vi "Acquire Data using Metronome - cRIO.vi"() -> ()   [LabVIEW 2010]
uses:
  <vilib>/eio/EIONode/EIONode.xnode
  <vilib>/rvi/eio/nirviEIOImplementation/nirviEIOImplementation.xnode
  <vilib>/rvi/eio/common/nirviEmuClasses.ctl
  <vilib>/rvi/eio/common/nirviEmuTemplateMethod_noerrors.vi
  FPGA Timekeeper.lvlib
panel:
  out "sample timestamp (ns)":u64
  out "Mod1/AI0":fxp<+/-,20,5>
  in  "loop period (ns)":u32=1000000000
  in  "start time (ns)":u64
  out "offset from time reference":i32
  out "FPGA Timekeeper locked":bool
  out "FPGA Timekeeper time (ns)":u64
  # "This example samples an analog input using the Metronome VI of the FPGA Timekeeper API."
  # "Analog Sampling Info"
  # "The default values for the controls  loop period (ns), and start time (ns) will sample an analog input at the rate of 1 Hz with each sample aligned to the beginning of each second."
  # "Acquired Data"
  # "Analog input modules need time to perform the conversion.  The difference in time between when the start of the conversion and the sample timestamp is the conversion time."
  # "FPGA Timekeeper"
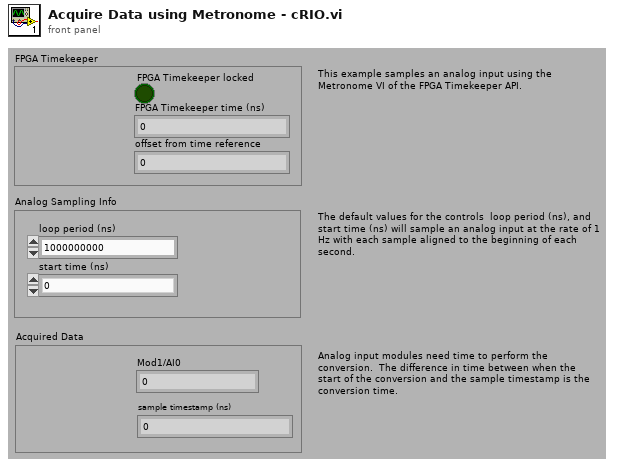
[diagram p1: front panel]
types:
  T1 = typedef "nirviEmuClasses.ctl" = enum16{"IO Read", "IO Write", "Method", "Property Read", "Property Write"}
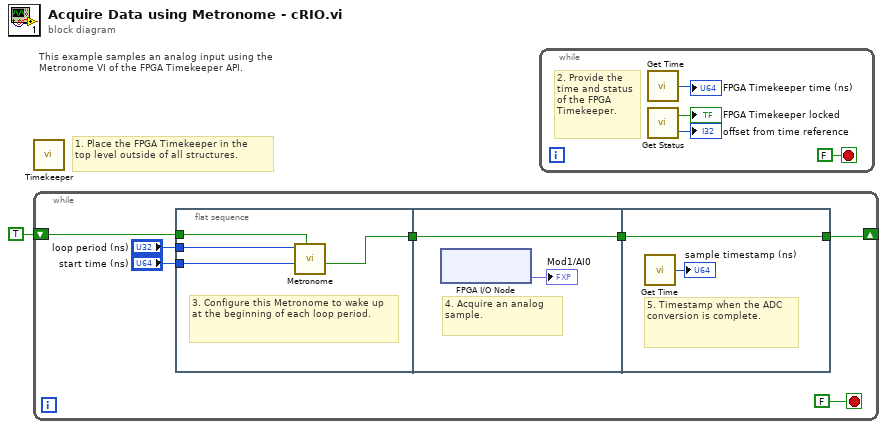
[diagram p0: block diagram]
diagram:
  # "This example samples an analog input using the Metronome VI of the FPGA Timekeeper API."
  # "1. Place the FPGA Timekeeper in the\ntop level outside of all structures."
  n1 = call "Timekeeper.vi"() -> ()  [unwired: 12 in]
  n2 = while {
    shift-right: [w7] -> _
    shift-left: TRUE ("Time Snapped Event") -> [w8]
    stop <- FALSE stop-if-true
    n3 = flat-sequence {
      tunnel: w8 -> [w12]
      tunnel: "start time (ns)" -> [w10]
      tunnel: "loop period (ns)" -> [w11]
      tunnel: [w9] -> w3
      tunnel: w3 -> [w14]
      tunnel: [w14] -> w2
      tunnel: [w35] -> w7
      tunnel: w2 -> [w35]
      frame #0 {
        # "3. Configure this Metronome to wake up at the beginning of each loop period."
        n4 = call "Metronome.vi"("initialize"=w12, "start time (ns)"=w10, "loop period (ns)"=w11) -> ("time snapped event"=w9:bool)  [unwired: 5 in, 1 out]
      }
      frame #1 {
        # "4. Acquire an analog sample."
        n5 = xnode "FPGA I/O Node"() -> ("Mod1/AI0"=→"Mod1/AI0":fxp<+/-,20,5>)  [unwired: 1 in, 1 out]
      }
      frame #2 {
        # "5. Timestamp when the ADC conversion is complete."
        n6 = call "Get Time.vi"() -> ("time (ns)"=→"sample timestamp (ns)":u64)
      }
    }
  }
  n7 = while {
    stop <- FALSE stop-if-true
    # "2. Provide the time and status of the FPGA Timekeeper."
    n8 = call "Get Time.vi"() -> ("time (ns)"=→"FPGA Timekeeper time (ns)":u64)
    n9 = call "Get Status.vi"() -> ("FPGA Timekeeper locked"=→"FPGA Timekeeper locked":bool, "offset from time reference"=→"offset from time reference":i32)
  }
